vi "Audit Trail.vi"(8 "error in":errorcluster, 10 "connection reference":T1, 11 "Event":string) -> (0 "error IO":errorcluster)   [LabVIEW 2018]
uses:
  <vilib>/addons/database/Connection.llb/Conn ObjectReference.ctl
  <vilib>/addons/database/Auxilliary.llb/DB Tools Cursor Type.ctl
  Host Globals/Global 1.vi
  <vilib>/addons/database/Connection.llb/Conn Execute.vi
  <vilib>/addons/database/Recordset.llb/Rec Destroy - Connection.vi
  <vilib>/addons/database/NI_Database_API.lvlib
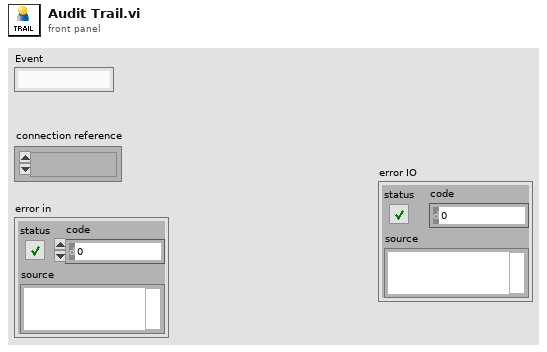
[diagram p1: front panel]
types:
  T1 = typedef "NI_Database_API.lvlib/Conn ObjectReference.ctl" = refnum<k1>
  T2 = typedef "NI_Database_API.lvlib/DB Tools Cursor Type.ctl" = enum16{"forward-only", "keyset", "dynamic", "static"}
  T3 = typedef "NI_Database_API.lvlib/Rec ObjectReference.ctl" = refnum<k1>
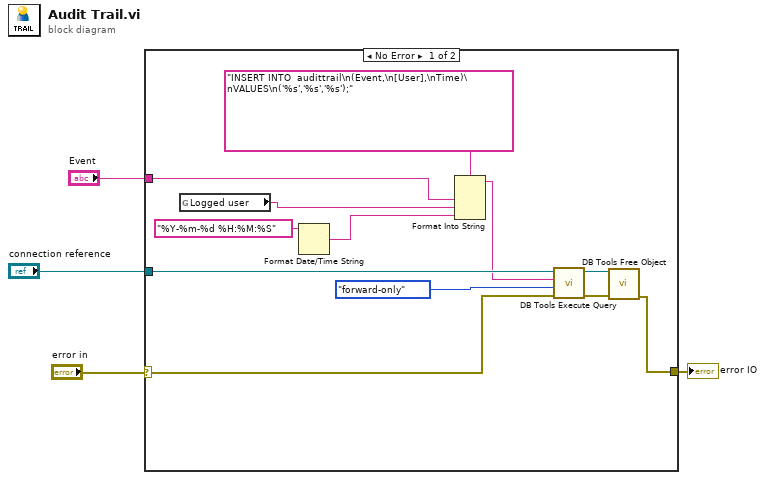
[diagram p0: block diagram]
diagram:
  n1 = case shown="No Error" "error in" {
    selector: "error in" -> [w16 w17]
    tunnel: "Event" -> [w13 _]
    tunnel: [w8 w17] -> w2
    tunnel: "connection reference" -> [w15 _]
    frame No Error {
      n2 = global read "Global 1.vi" "Logged user"() -> (w6:string)
      n3 = Format Date/Time String(time format string (%c)="%Y-%m-%d %H:%M:%S") -> (date/time string=w12:string)  [unwired: 2 in]
      n4 = Format Into String(format string="INSERT INTO  audittrail\n(Event,\n[User],\nTime)\nVALUES\n('%s','%s','%s');", w13, w6, w12) -> (resulting string=w11:string)  [unwired: 2 in, 1 out]
      n5 = call-poly <vilib>:"DB Tools Execute Query.vi"("error in (no error)"=w16, "cursor type"=DB_Tools_Cursor_Type."forward-only", "SQL query"=w11, "connection reference"=w15) -> ("error out"=w10:errorcluster, "recordset reference"=w9:T3)  [unwired: 4 in]
      n6 = call-poly <vilib>:"DB Tools Free Object.vi"("error in (no error)"=w10, "recordset reference"=w9) -> ("error out"=w8:errorcluster)  [unwired: 8 in, 1 out]
    }
    frame Error {
    }
  }
  "error IO" <- w2
